vi "sort polymorphs.vi"() -> ()   [LabVIEW 2013, in "scripting tools.lvlib"]
uses:
  scripting tools.lvlib
panel:
  in  "order":string[](array[string])
  in  "PolyVI Refnum":refnum<vi>
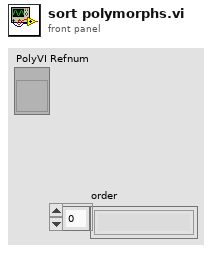
[diagram p1: front panel]
types:
  T1 = cluster{"VIPath":path, "Menu Name":string, "Selector Name":string}[]
  T2 = cluster{"VIPath":path, "Menu Name":string, "Selector Name":string}
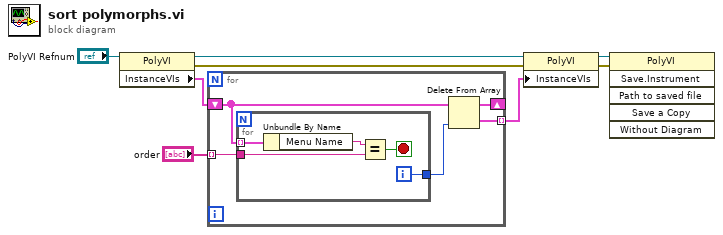
[diagram p0: block diagram]
diagram:
  n1 = property class="PolyVI"(reference="PolyVI Refnum") -> (reference out=w8:refnum<vi>, error out=w5:errorcluster, "InstanceVIs"=w4:T1)  [unwired: 1 in]
  n2 = for {
    shift-right: [w12] -> _
    shift-left: w4 -> [w13]
    tunnel: [w10] -> w3 mode=indexing
    tunnel: "order" -> [w9] mode=indexing
    n3 = for {
      tunnel: w13 -> [w18] mode=indexing
      tunnel: w9 -> [w16]
      tunnel: [w14] -> w11
      i -> [w14]
      stop <- w15 stop-if-true
      n4 = Unbundle By Name(w18) -> ("Menu Name"=w17:string)
      n5 = Equal?(x=w17, y=w16) -> (x = y?=w15:bool)
    }
    n6 = Delete From Array(array=w13, index=w11) -> (deleted portion=w10:T2, array with subset deleted=w12:T1)  [unwired: 1 in]
  }
  n7 = property class="PolyVI"(reference=w8, error in=w5, "InstanceVIs"=w3) -> (reference out=w7:refnum<vi>, error out=w6:errorcluster)
  n8 = invoke class="PolyVI" method="Save.Instrument"(reference=w7, error in=w6) -> ()  [unwired: 4 in, 6 out]
